vi "Read_uCRegister.vi"(8 "error in":errorcluster, 9 "uC Address":i32=23, 10 "id_in":i32, 11 "connection ID in":refnum<k5>) -> (0 "error out":errorcluster, 1 "Register value":i32, 2 "id_out":i32, 3 "connection ID out":refnum<k5>, 5 "Data out":string)   [LabVIEW 2009]
doc: "This VI reads a specific uC register by doing some redundancy to assure that the reading is correct."
panel:
  out "Numeric":i32
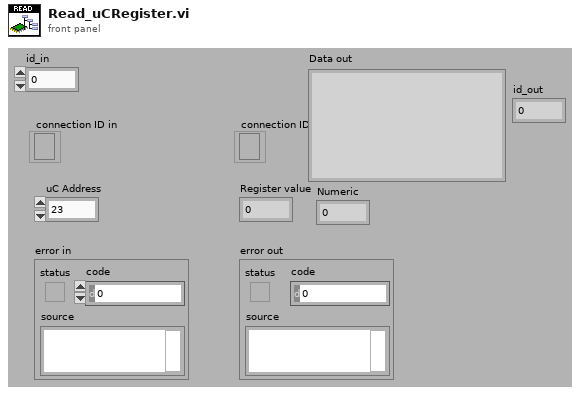
[diagram p1: front panel]
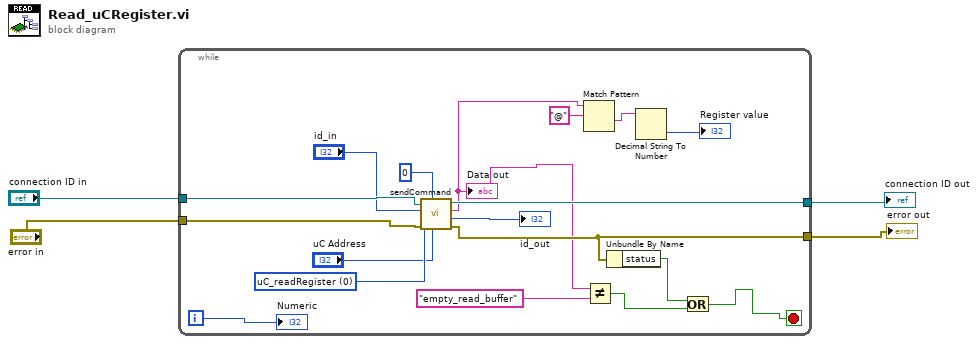
[diagram p0: block diagram]
diagram:
  n1 = while {
    tunnel: "connection ID in" -> [w22]
    tunnel: "error in" -> [w21]
    tunnel: [w13] -> w2
    tunnel: [w9] -> w1
    i -> [w11]
    stop <- w10 stop-if-true
    w16 = u16 0 items=["sendCommand"=9, "FPGA_writeRegister"=3, "FPGA_readRegister"=2, "uC_writeRegister"=1, "uC_readRegister"=0] ("Action")
    n2 = call "sendCommand.vi"("Address"="uC Address", "Data"=0, "error in"=w21, "Action"=w16, "id_in"="id_in", "connection ID"=w22) -> ("error out"=w9:errorcluster, "id_out"=→"id_out":i32, "Data out"=w6:string, "connection ID out"=w13:refnum<k5>)  [unwired: 1 in, 1 out]
    "Data out" <- w6
    n3 = Match Pattern(string=w6, regular expression="@" ("search string/char (-)")) -> (after substring=w19:string)  [unwired: 1 in, 3 out]
    n4 = Not Equal?(x=w6, y="empty_read_buffer") -> (x != y?=w7:bool)
    n5 = Unbundle By Name(w9) -> ("status"=w8:bool)
    n6 = Decimal String To Number(string=w19) -> (number=→"Register value":i32)  [unwired: 2 in, 1 out]
    n7 = Or(x=w8, y=w7) -> (x .or. y?=w10:bool)
    "Numeric" <- w11
  }
  "connection ID out" <- w2
  "error out" <- w1
